vi "ControlRoom-FPGA.vi"() -> ()   [LabVIEW 2016]
doc: "Fpga for Control room rio"
uses:
  <vilib>/Platform/TimedLoop/XDataNode/timing_clust.ctl
  <vilib>/Platform/TimedLoop/XDataNode/nitl_modes.ctl
  <vilib>/Platform/TimedLoop/XDataNode/wakeup.ctl
  <vilib>/rvi/FXPMathLib/basic elements/FxpIntAccumulator/subVIs/nifxpmath_IntAccumulator_SimConfig.ctl
  <vilib>/rvi/Emulation/niFpgaGetClockAttributes.vi
  <vilib>/rvi/Emulation/niFpgaSctlEmulationGetInTimedLoop.vi
  <vilib>/rvi/Emulation/niFpgaEmulationReportErrorSimple.vi
  <vilib>/rvi/eio/common/nirviEmuTemplateMethod_errors.vi
  <vilib>/rvi/Analysis/common/codeGenErrors/XNode/niFpgaXNodeCodeGenErrorHandle.vi
  <vilib>/rvi/Emulation/niFpgaCriticalErrorInLSC.vi
  <vilib>/rvi/FXPMathLib/basic elements/FxpIntAccumulator/simVIs/DllFxpIntAccumulator_sub.vi
  <vilib>/eio/EIONode/EIONode.xnode
  <vilib>/rvi/Analysis/measure/dc-rms/XNode/niFpgaDC-RMS.xnode
  <vilib>/Platform/TimedLoop/XDataNode/XDataNode.xnode
  <vilib>/rvi/FXPMathLib/basic elements/FxpIntAccumulator/XNode/nifxpmath_IntAccumulator.xnode
  <vilib>/rvi/FXPMathLib/FxpMul/XNode/nifxpmath_Multiplier.xnode
  <vilib>/Platform/TimedLoop/XDataNode/XDNodeRunTimeDep.lvlib
  <vilib>/rvi/FXPMathLib/sim/FxpSim.dll
panel:
  out "terminal voltage":fxp<+/-,26,5> format="%.23g"
  out "Terminal readbacks":fxp<+/-,26,5>[](array[numeric]) format="%.23g"
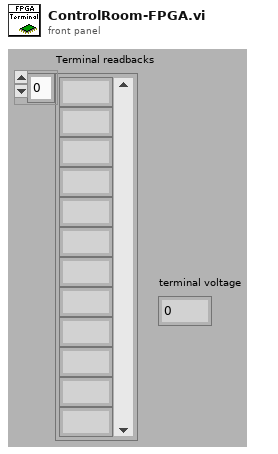
[diagram p1: front panel]
types:
  T1 = typedef "XDNodeRunTimeDep.lvlib/timing_clust.ctl" = cluster{"Expected End [f-1]":u64, "Actual End [f-1]":u64, "Finished Late? [f-1]":bool, "Expected End [i-1]":u64, "Actual End [i-1]":u64, "Finished Late? [i-1]":bool, "Expected Start [i]":u64, "Actual Start [i]":u64, "Expected Start [f]":u64, "Actual Start [f]":u64, "Source Name":string, "Structure Name":string, "Period":i64, "Deadline":i64, "Offset":i64, "Start":i64, "Priority":i32, "Timeout":i32, "Mode":T2, "Wakeup Reason":T3, "Error":errorcluster, "Source Type":string, "Secondary Source Type":string, "Global End Time":u64, "Global Start Time":u64, "Frame Duration":u64, "Iteration Duration":u64, "Assigned CPU":i32, "I/O Scan Engine Mode":u32}
  T2 = typedef "XDNodeRunTimeDep.lvlib/nitl_modes.ctl" = enum32{"No Change", "Process missed periods, maintain original phase", "Discard missed periods, maintain original phase", "Process missed periods, ignore original phase", "Discard missed periods, ignore original phase"}
  T3 = typedef "XDNodeRunTimeDep.lvlib/wakeup.ctl" = enum32{"Normal", "Aborted", "Asynchronous wakeup", "Timing source error", "Timed loop error", "Timeout"}
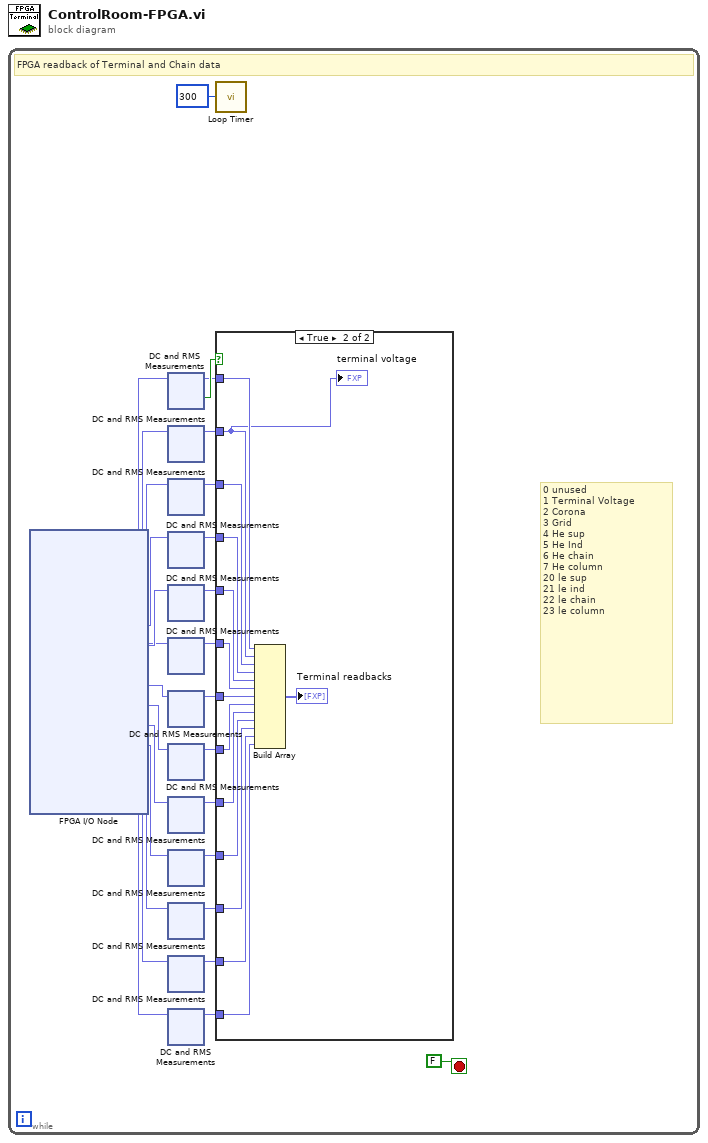
[diagram p0: block diagram]
diagram:
  n1 = while {
    stop <- FALSE stop-if-true
    # "0 unused\n1 Terminal Voltage\n2 Corona\n3 Grid\n4 He sup\n5 He Ind\n6 He chain\n7 He column\n20 le sup\n21 le ind\n22 le chain\n23 le column"
    # "FPGA readback of Terminal and Chain data"
    n2 = xnode "FPGA I/O Node"() -> ("Mod5/AI0"=w27:fxp<+/-,26,5>, "Mod5/AI1"=w24:fxp<+/-,26,5>, "Mod5/AI2"=w23:fxp<+/-,26,5>, "Mod5/AI3"=w22:fxp<+/-,26,5>, "Mod5/AI4"=w21:fxp<+/-,26,5>, "Mod5/AI5"=w20:fxp<+/-,26,5>, "Mod5/AI6"=w14:fxp<+/-,26,5>, "Mod5/AI7"=w12:fxp<+/-,26,5>, "Mod5/AI17"=w10:fxp<+/-,26,5>, "Mod5/AI18"=w8:fxp<+/-,26,5>, "Mod5/AI19"=w6:fxp<+/-,26,5>, "Mod5/AI20"=w4:fxp<+/-,26,5>, "Mod5/AI16"=w2:fxp<+/-,26,5>)  [unwired: 13 in, 13 out]
    n3 = xnode "DC and RMS Measurements"("input data"=w27) -> ("DC"=w25:fxp<+/-,26,5>, "output valid"=w26:bool)  [unwired: 1 in]
    n4 = xnode "DC and RMS Measurements"("input data"=w24) -> ("DC"=w19:fxp<+/-,26,5>)  [unwired: 1 in, 1 out]
    n5 = xnode "DC and RMS Measurements"("input data"=w23) -> ("DC"=w18:fxp<+/-,26,5>)  [unwired: 1 in, 1 out]
    n6 = xnode "DC and RMS Measurements"("input data"=w22) -> ("DC"=w17:fxp<+/-,26,5>)  [unwired: 1 in, 1 out]
    n7 = xnode "DC and RMS Measurements"("input data"=w21) -> ("DC"=w16:fxp<+/-,26,5>)  [unwired: 1 in, 1 out]
    n8 = xnode "DC and RMS Measurements"("input data"=w20) -> ("DC"=w15:fxp<+/-,26,5>)  [unwired: 1 in, 1 out]
    n9 = xnode "DC and RMS Measurements"("input data"=w14) -> ("DC"=w13:fxp<+/-,26,5>)  [unwired: 1 in, 1 out]
    n10 = xnode "DC and RMS Measurements"("input data"=w12) -> ("DC"=w11:fxp<+/-,26,5>)  [unwired: 1 in, 1 out]
    n11 = xnode "DC and RMS Measurements"("input data"=w10) -> ("DC"=w9:fxp<+/-,26,5>)  [unwired: 1 in, 1 out]
    n12 = xnode "DC and RMS Measurements"("input data"=w8) -> ("DC"=w7:fxp<+/-,26,5>)  [unwired: 1 in, 1 out]
    n13 = xnode "DC and RMS Measurements"("input data"=w6) -> ("DC"=w5:fxp<+/-,26,5>)  [unwired: 1 in, 1 out]
    n14 = xnode "DC and RMS Measurements"("input data"=w4) -> ("DC"=w3:fxp<+/-,26,5>)  [unwired: 1 in, 1 out]
    n15 = xnode "DC and RMS Measurements"("input data"=w2) -> ("DC"=w1:fxp<+/-,26,5>)  [unwired: 1 in, 1 out]
    n16 = call "Loop Timer"("Count(uSec)"=u32 300 ("Count(Ticks)")) -> ()  [unwired: 1 out]
    n17 = case shown="True" w26 {
      tunnel: w25 -> [_ w1082]
      tunnel: w19 -> [_ w1070]
      tunnel: w18 -> [_ w1081]
      tunnel: w17 -> [_ w1080]
      tunnel: w16 -> [_ w1079]
      tunnel: w15 -> [_ w1078]
      tunnel: w13 -> [_ w1077]
      tunnel: w11 -> [_ w1076]
      tunnel: w9 -> [_ w1075]
      tunnel: w7 -> [_ w1074]
      tunnel: w5 -> [_ w1073]
      tunnel: w3 -> [_ w1072]
      tunnel: w1 -> [_ w1071]
      frame False {
      }
      frame True {
        n18 = Build Array(w1082, w1070, w1081, w1080, w1079, w1078, w1077, w1076, w1075, w1074, w1073, w1072, w1071) -> (→"Terminal readbacks":fxp<+/-,26,5>[])
        "terminal voltage" <- w1070
      }
    }
  }
